vi "배열 내림차순으로 재배열 (차선 라이다 통합).vi"(9 "내림차순 기준 인덱스":i32, 10 "행 수":i32, 11 "입력 배열":dbl[][](array[numeric])) -> (3 "출력 배열":dbl[][](array[numeric]))   [LabVIEW 2016]
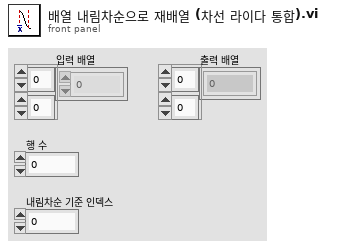
[diagram p1: front panel]
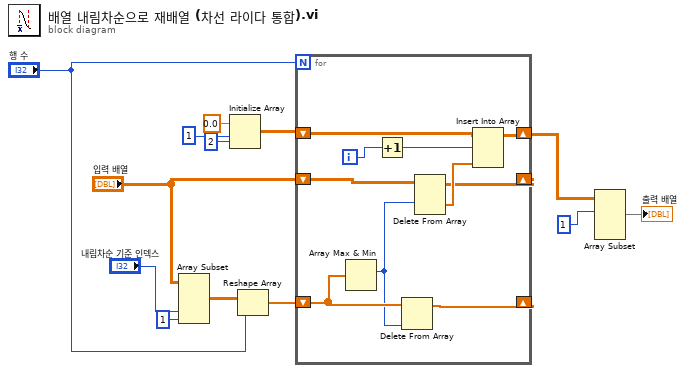
[diagram p0: block diagram]
diagram:
  n1 = Array Subset(array="입력 배열", index (col)="내림차순 기준 인덱스", length (col)=1 ("길이")) -> (w10:dbl[][])  [unwired: 2 in]
  n2 = Initialize Array(0.0 ("원소"), 1 ("차원 크기"), 2 ("차원 크기")) -> (w3:dbl[][])
  n3 = Reshape Array(w10, "행 수") -> (w9:dbl[])
  n4 = for {
    N: "행 수" -> [_]
    shift-right: [w14] -> _
    shift-left: "입력 배열" -> [w21]
    shift-right: [w15] -> w2
    shift-left: w3 -> [w18]
    shift-right: [w22] -> _
    shift-left: w9 -> [w23]
    i -> [w17]
    n5 = Array Max & Min(array=w23) -> (max index (indices)=w20:i32)  [unwired: 3 out]
    n6 = Increment(x=w17) -> (x+1=w16:i32)
    n7 = Delete From Array(array=w23, index=w20) -> (array with subset deleted=w22:dbl[])  [unwired: 1 in, 1 out]
    n8 = Delete From Array(array=w21, index (row)=w20) -> (deleted portion=w19:dbl[], array with subset deleted=w14:dbl[][])  [unwired: 2 in]
    n9 = Insert Into Array(array=w18, index (row)=w16, new element=w19) -> (w15:dbl[][])  [unwired: 1 in]
  }
  n10 = Array Subset(array=w2, index (row)=1 ("인덱스")) -> (→"출력 배열":dbl[][])  [unwired: 3 in]
